vi "MIMO Rx Streaming Multi-Channel (Host).vi"() -> ()   [LabVIEW 2013]
doc: "This template is for the Simple NI-USRP Streaming design, a design that shows the basics of streaming data from an NI 294x/295x device. Refer to the block diagram for more information about how to use this template."
uses:
  <vilib>/userdefined/Silver/nirio_resource_slv.ctl
  SubVIs/Start Trigger.ctl
  <vilib>/Utility/error.llb/DialogType.ctl
  SubVIs/Configure Signal (Level).vi
panel:
  in  "number of samples is finite":bool=TRUE
  in  "reference level rf 1":dbl caption="Reference Level" format="%#_gdBm"
  in  "reference level rf 0":dbl caption="Reference Level" format="%#_gdBm"
  in  "lo frequency rf 1":dbl=-1.0 caption="LO Frequency" format="%#.3pHz"
  in  "lo frequency rf 0":dbl=-1.0 caption="LO Frequency" format="%#.3pHz"
  in  "frequency rf 1":dbl=2000000000.0 caption="Frequency" format="%#.3pHz"
  in  "frequency rf 0":dbl=2000000000.0 caption="Frequency" format="%#.3pHz"
  in  "antenna rf 1":string(combo)="RX1" caption="Active Antenna"
  in  "antenna rf 0":string(combo)="RX1" caption="Active Antenna"
  in  "enable rf 1":bool=TRUE
  in  "enable rf 0":bool=TRUE
  in  "USRP RIO devices":T1[](array[typedef])=["RIO0", "RIO1"] caption="USRP RIO Devices"
  in  "reference frequency source":string(combo)="REF IN" caption="Reference Frequency Source"
  in  "sample rate":dbl=10000000.0 caption="Sample Rate" format="%#.3pS/s"
  in  "start trigger":T2=enum."Immediate" caption="Start Trigger"
  in  "tab control":T3(tab)
  out "Power Spectrum":cluster{"f0":dbl, "df":dbl, "magnitude":dbl[]}[](graph)
  out "Power Level":dbl[][](graph)
  out "I & Q Data":dbl[][](graph)
  in  "number of samples":u32=8192 caption="Number of Samples"
  in  "stop":bool
  # "Multi-Channel MIMO Rx Streaming"
  # "This template is for the Simple NI-USRP Streaming design, a design that shows the basics of streaming data from an NI 294x/295x device. See the block diagram for more information on how to use this template."
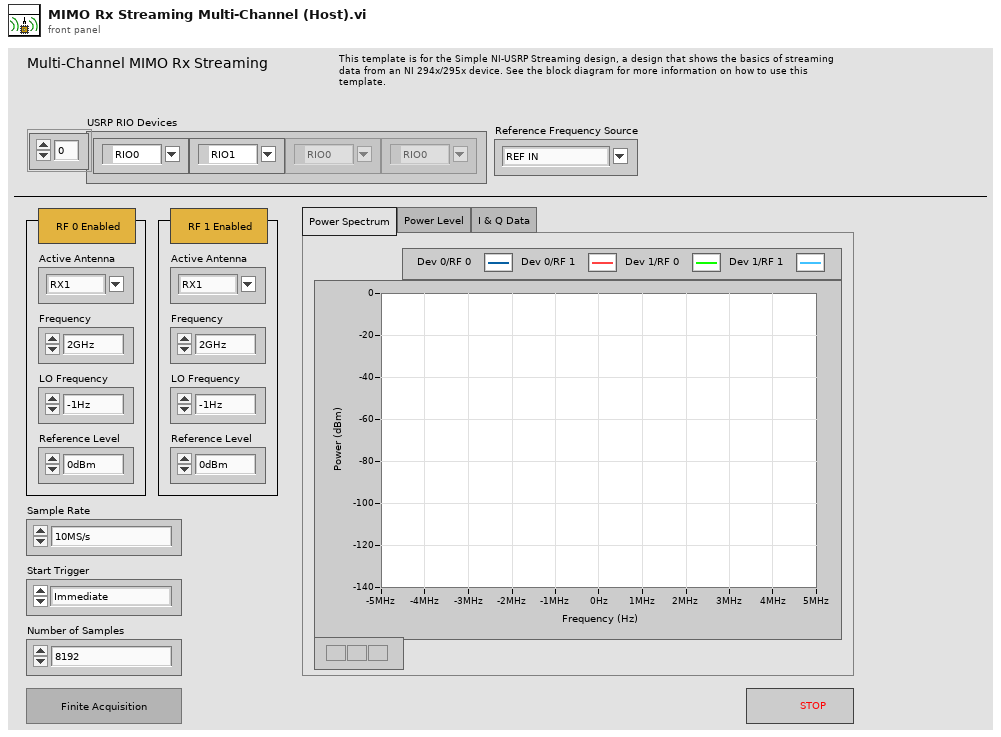
[diagram p1: front panel]
types:
  T1 = typedef "nirio_resource_slv.ctl" = tag
  T2 = typedef "Start Trigger.ctl" = enum8{"Software", "Digital Edge", "Rx Start Trigger", "Tx Start Trigger", "Immediate"}
  T3 = enum32{"Power Spectrum", "Power Level", "I & Q Data"}
  T4 = typedef "DialogType.ctl" = u16
  T5 = typedef "niUsrpRio Config v1 Host.lvlib/niUsrpRio Session.ctl" = cluster{"Global Settings Register Bus":T6, "Radio 0 Settings Register Bus":T6, "Rx NI-USRP session":refnum<k15>, "Tx NI-USRP session":refnum<k15>, "FPGA Interface":refnum<k20>, "RIO Interface Number":u32, "EEPROM Header":T7, "Device Data Header":T8, "EEPROM Characterization Header":T9, "Characterization Data":T10[], "Characterization Data Valid?":bool, "Radio 1 Settings Register Bus":T6, "Radio Settings Bus Semaphore":T12}
  T6 = typedef "niInstr Register Bus v0 Host.lvlib/Register Bus Session.ctl" = refnum<queue>
  T7 = typedef "niUsrpRio Config v1 Host.lvlib/EEPROM Header.ctl" = cluster{"Checksum":u32, "Product Code":u16, "Hardware Current Version":u16, "Hardware Oldest Compatible Version":u16, "EEPROM Map Current Version":u16, "EEPROM Map Oldest Compatible Version":u16, "User Password":string, "Pointer to Factory Header":u32, "Pointer to User Header":u32, "Recommended Interval":u16, "Number of Reserved Bytes":i32, "Number of Daughterboards":u8, "Daughterboard IDs":u16[], "Daughterboard Serial Numbers":string[]}
  T8 = typedef "niUsrpRio Config v1 Host.lvlib/EEPROM Device Data Header.ctl" = cluster{"Checksum":u32, "Number of Channels":u8, "Number of Gain Settings":u16[], "Pointer to Characterization Data":u32[], "Number of Reserved Bytes":i32, "Number of Frequencies":u16[]}
  T9 = typedef "niUsrpRio Config v1 Host.lvlib/EEPROM Characterization Header.ctl" = cluster{"Checksum":u32, "Date":timestamp, "Temperature":sgl, "Misc. Info":string, "Pointer to Device Data Header":u32, "Number of Reserved Bytes":i32}
  T10 = typedef "niUsrpRio Config v1 Host.lvlib/Characterization Data.ctl" = cluster{"Gains[dB]":dbl[], "Frequencies [Hz]":dbl[], "IQ Imbalance Table":T11[], "Measured Gains[dB]":dbl[][]}
  T11 = typedef "niUsrpRio Config v1 Host.lvlib/IQ Imbalance.ctl" = cluster{"Gain Imbalance [linear]":dbl, "Phase Imbalance [radians]":dbl, "Offset":cdb}
  T12 = typedef "Semaphore RefNum" = refnum<k1>
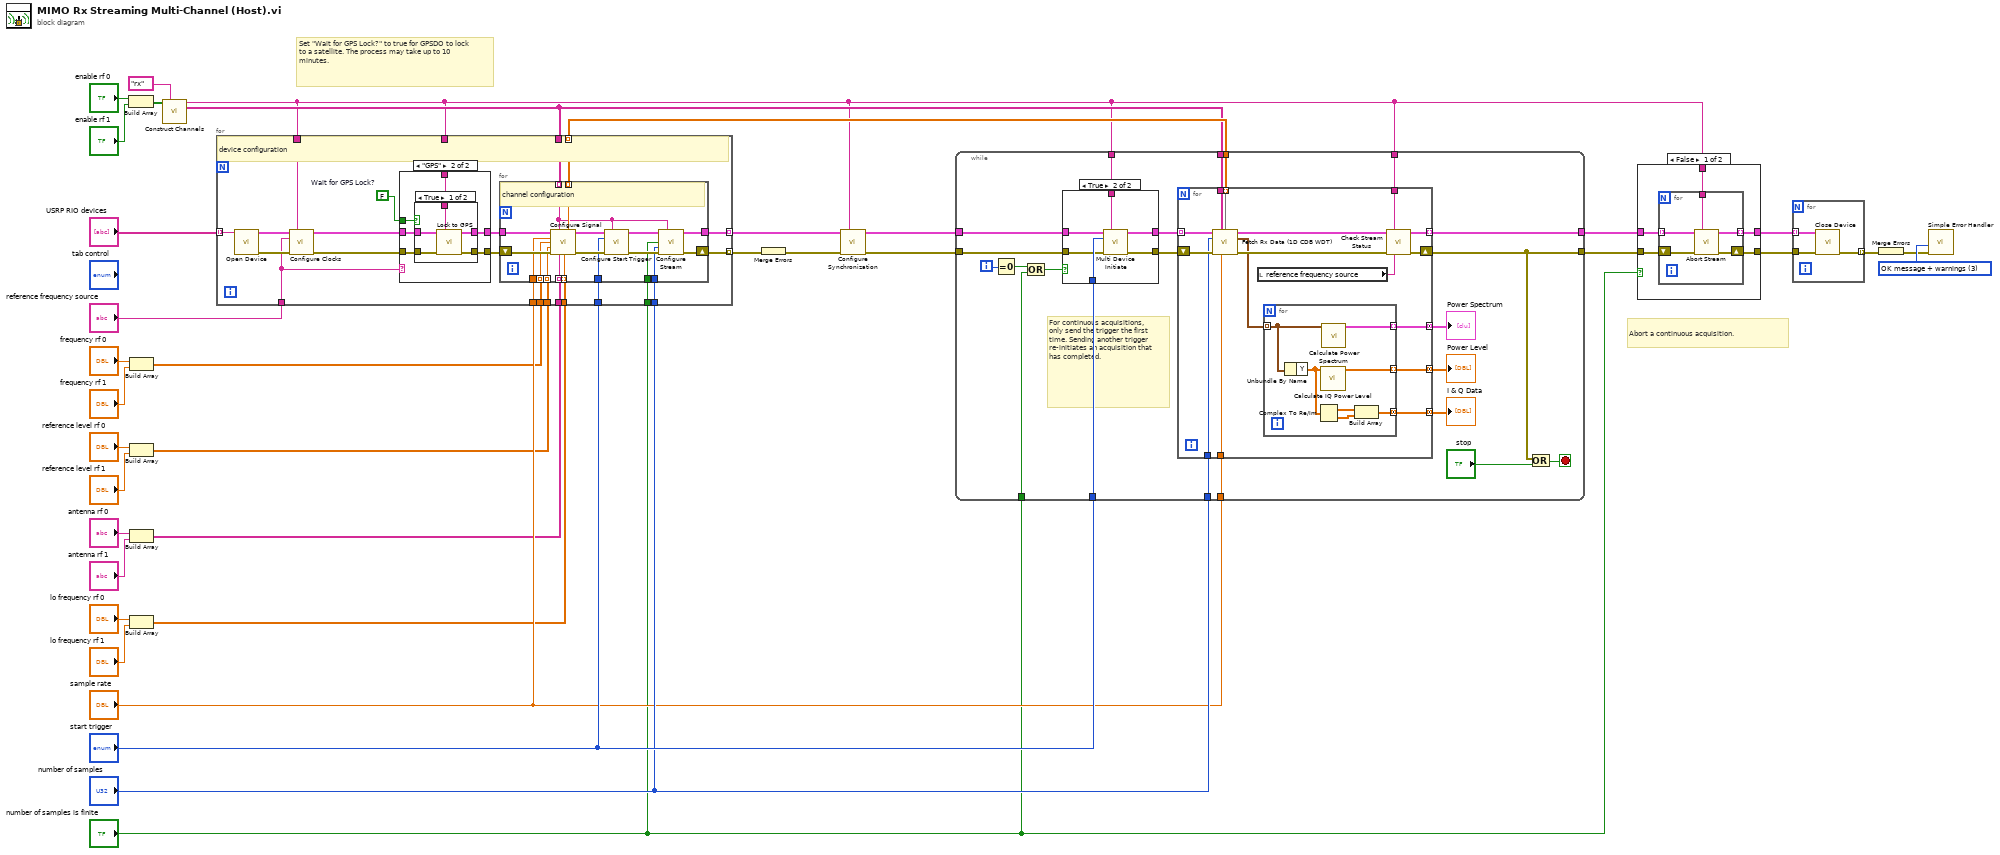
[diagram p0: block diagram]
diagram:
  w35 = T4 3 items=["no dialog", "OK message", "continue or stop message", "OK message + warnings", "continue/stop + warnings"] ("type of dialog (OK msg:1)")
  # "Set \"Wait for GPS Lock?\" to true for GPSDO to lock to a satellite. The process may take up to 10 minutes."
  # "Abort a continuous acquisition."
  n1 = Build Array("enable rf 0", "enable rf 1") -> (w15:bool[])
  n2 = Build Array("frequency rf 0", "frequency rf 1") -> (w5:dbl[])
  n3 = Build Array("reference level rf 0", "reference level rf 1") -> (w6:dbl[])
  n4 = Build Array("antenna rf 0", "antenna rf 1") -> (w14:string[])
  n5 = Build Array("lo frequency rf 0", "lo frequency rf 1") -> (w9:dbl[])
  n6 = call "Construct Channels.vi"("enabled channels"=w15, "scope"="rx") -> ("scope"=w1:string, "channels"=w3:string[])  [unwired: 12 in]
  n7 = for {
    tunnel: [w60] -> w37 mode=indexing
    tunnel: [w59] -> w34 mode=indexing
    tunnel: "start trigger" -> [w58]
    tunnel: [w55] -> w32 mode=indexing
    tunnel: "number of samples" -> [w54]
    tunnel: "number of samples is finite" -> [w53]
    tunnel: "reference frequency source" -> [w39]
    tunnel: w9 -> [w52]
    tunnel: w5 -> [w51]
    tunnel: w6 -> [w50]
    tunnel: w3 -> [w49]
    tunnel: "sample rate" -> [w48]
    tunnel: "USRP RIO devices" -> [w47] mode=indexing
    tunnel: w14 -> [w46]
    tunnel: w1 -> [w45]
    tunnel: w1 -> [w38]
    w44 = FALSE  # Wait for GPS Lock?
    # "device configuration"
    n8 = call "Open Device.vi"("USRP RIO device"=w47) -> ("niUsrpRio Session (out)"=w57:T5, "error out"=w56:errorcluster)  [unwired: 13 in]
    n9 = call "Configure Clocks.vi"("niUsrpRio Session"=w57, "scope"=w45, "Reference Frequency Source"=w39, "error in"=w56) -> ("niUsrpRio Session (out)"=w41:T5, "error out"=w42:errorcluster)  [unwired: 10 in]
    n10 = case shown="\"GPS\"" w39 {
      tunnel: w41 -> [w62 w68]
      tunnel: [w62 w67] -> w40
      tunnel: [w61 w66] -> w43
      tunnel: w42 -> [w61 w65]
      tunnel: w38 -> [_ w64]
      tunnel: w44 -> [_ w63]
      frame Default {
      }
      frame "GPS" {
        n11 = case shown="True" w63 {
          tunnel: w68 -> [w70 w75]
          tunnel: [w73 w75] -> w67
          tunnel: [w72 w74] -> w66
          tunnel: w65 -> [w69 w74]
          tunnel: w64 -> [w71 _]
          frame True {
            n12 = call "Lock to GPS.vi"("niUsrpRio Session"=w70, "scope"=w71, "error in"=w69) -> ("niUsrpRio Session (out)"=w73:T5, "error out"=w72:errorcluster)  [unwired: 11 in]
          }
          frame False {
          }
        }
      }
    }
    n13 = for {
      tunnel: [w91] -> w59
      tunnel: w58 -> [w90]
      tunnel: w40 -> [w85]
      tunnel: [w84] -> w55 mode=indexing
      tunnel: w54 -> [w83]
      tunnel: w53 -> [w82]
      shift-right: [w92] -> w60
      shift-left: w43 -> [w86]
      tunnel: w49 -> [w81] mode=indexing
      tunnel: w52 -> [w80] mode=indexing
      tunnel: w51 -> [w79] mode=indexing
      tunnel: w50 -> [w78] mode=indexing
      tunnel: w48 -> [w77]
      tunnel: w46 -> [w76] mode=indexing
      # "channel configuration"
      n14 = call-poly "Configure Signal.vi"("niUsrpRio Session"=w85, "scope"=w81, "sample rate [S/s]"=w77, "frequency [Hz]"=w79, "level [dBm]"=w78, "error in"=w86, "Active Antenna"=w76, "LO frequency [Hz]"=w80) -> ("coerced vertical range [Vpp]"=w84:dbl, "niUsrpRio Session (out)"=w88:T5, "error out"=w93:errorcluster)  [unwired: 1 in, 4 out]
      n15 = call "Configure Start Trigger.vi"("niUsrpRio Session"=w88, "scope"=w81, "start trigger"=w90, "error in"=w93) -> ("niUsrpRio Session (out)"=w87:T5, "error out"=w89:errorcluster)  [unwired: 10 in]
      n16 = call "Configure Stream.vi"("niUsrpRio Session"=w87, "scope"=w81, "number of samples is finite"=w82, "number of samples"=w83, "error in"=w89) -> ("niUsrpRio Session (out)"=w91:T5, "error out"=w92:errorcluster)  [unwired: 9 in]
    }
  }
  n17 = Merge Errors(w37) -> (w23:errorcluster)
  n18 = call "Configure Synchronization.vi"("niUsrpRio Sessions"=w34, "scope"=w1, "error in"=w23) -> ("niUsrpRio Sessions (out)"=w21:T5[], "error out"=w22:errorcluster)  [unwired: 11 in]
  n19 = while {
    tunnel: w21 -> [w106]
    tunnel: [w113] -> w30
    tunnel: w32 -> [w99]
    tunnel: "sample rate" -> [w104]
    tunnel: "number of samples" -> [w103]
    tunnel: "start trigger" -> [w109]
    tunnel: w22 -> [w108]
    tunnel: [w112] -> w29
    tunnel: "number of samples is finite" -> [w100]
    tunnel: w3 -> [w98]
    tunnel: w1 -> [w95]
    tunnel: w1 -> [w94]
    i -> [w101]
    stop <- w115 stop-if-true
    # "For continuous acquisitions, only send the trigger the first time. Sending another trigger re-initiates an acquisition that has completed."
    # "Acquire and Fetch a waveform"
    n20 = Equal To 0?(x=w101) -> (x = 0?=w102:bool)
    n21 = Or(x=w102, y=w100) -> (x .or. y?=w96:bool)
    n22 = case shown="True" w96 {
      tunnel: w109 -> [_ w123]
      tunnel: w108 -> [w117 w122]
      tunnel: [w117 w121] -> w107
      tunnel: w106 -> [w116 w120]
      tunnel: [w116 w119] -> w105
      tunnel: w94 -> [_ w118]
      frame False {
      }
      frame True {
        n23 = call "Multi Device Initiate.vi"("niUsrpRio Sessions"=w120, "scope"=w118, "start trigger"=w123, "error in"=w122) -> ("niUsrpRio Sessions (out)"=w119:T5[], "error out"=w121:errorcluster)  [unwired: 10 in]
      }
    }
    n24 = for {
      tunnel: [w139] -> w113 mode=indexing
      tunnel: [w137] -> w111 mode=concatenating
      tunnel: [w136] -> w110 mode=concatenating
      tunnel: w105 -> [w134] mode=indexing
      tunnel: w104 -> [w131]
      tunnel: w103 -> [w130]
      tunnel: w99 -> [w129] mode=indexing
      tunnel: w98 -> [w128]
      tunnel: [w126] -> w97 mode=concatenating
      shift-right: [w138] -> w112
      shift-left: w107 -> [w135]
      tunnel: w95 -> [w125]
      n25 = call "Fetch Rx Data (1D CDB WDT).vi"("niUsrpRio Session"=w134, "scope"=w128, "vertical ranges [Vpp]"=w129, "number of samples"=w130, "error in"=w135, "sample rate"=w131) -> ("niUsrpRio Session (out)"=w132:T5, "Waveforms (CDB WDT)"=w127:waveform(cdb)[], "error out"=w133:errorcluster)  [unwired: 7 in]
      n26 = local read "reference frequency source"() -> (w124:string)
      n27 = for {
        tunnel: [w146] -> w137 mode=indexing
        tunnel: [w145] -> w136 mode=concatenating
        tunnel: w127 -> [w140] mode=indexing
        tunnel: [w141] -> w126 mode=indexing
        n28 = Unbundle By Name(w140) -> ("Y"=w144:cdb[])
        n29 = Complex To Re/Im(x + iy=w144) -> (x=w143:dbl[], y=w142:dbl[])
        n30 = call "Calculate IQ Power Level.vi"("IQ data"=w144) -> ("power level (dBm)"=w146:dbl[])  [unwired: 14 in]
        n31 = call "Calculate Power Spectrum.vi"("IQ Waveform"=w140) -> ("power spectrum (dBm)"=w141:cluster{"f0":dbl, "df":dbl, "magnitude":dbl[]})  [unwired: 14 in]
        n32 = Build Array(w143, w142) -> (w145:dbl[][])
      }
      n33 = call "Check Stream Status.vi"("niUsrpRio Session"=w132, "scope"=w125, "error in"=w133, "reference frequency source"=w124) -> ("niUsrpRio Session (out)"=w139:T5, "error out"=w138:errorcluster)  [unwired: 9 in, 1 out]
    }
    "Power Level" <- w111
    "Power Spectrum" <- w97
    "I & Q Data" <- w110
    n34 = Or(x=w112, y="stop") -> (x .or. y?=w115:bool)
  }
  n35 = case shown="False" "number of samples is finite" {
    tunnel: w30 -> [w151 w158]
    tunnel: w29 -> [w150 w157]
    tunnel: [w149 w158] -> w28
    tunnel: [w148 w157] -> w27
    tunnel: w1 -> [w147 _]
    frame False {
      n36 = for {
        tunnel: w151 -> [w156] mode=indexing
        tunnel: [w155] -> w149 mode=indexing
        shift-right: [w153] -> w148
        shift-left: w150 -> [w154]
        tunnel: w147 -> [w152]
        n37 = call "Abort Stream.vi"("niUsrpRio Session"=w156, "scope"=w152, "error in"=w154) -> ("niUsrpRio Session (out)"=w155:T5, "error out"=w153:errorcluster)  [unwired: 11 in]
      }
    }
    frame True {
    }
  }
  n38 = for {
    tunnel: [w161] -> w36 mode=indexing
    tunnel: w28 -> [w160] mode=indexing
    tunnel: w27 -> [w159]
    n39 = call "Close Device.vi"("niUsrpRio Session"=w160, "error in"=w159) -> ("error out"=w161:errorcluster)  [unwired: 13 in]
  }
  n40 = Merge Errors(w36) -> (w20:errorcluster)
  n41 = call <vilib>:"Simple Error Handler.vi"("type of dialog (OK msg:1)"=w35, "error in (no error)"=w20) -> ()  [unwired: 3 in, 5 out]
